vi "Send Tasks To Workers.vi"(8 "error in (no error)":errorcluster, 11 "BuildServer in":refnum<class "BuildServer.lvclass">) -> (0 "error out":errorcluster, 3 "BuildServer out":refnum<class "BuildServer.lvclass">)   [LabVIEW 2017, in "BuildServer.lvlib" / "BuildServer.lvclass"]
uses:
  BuildServer.lvclass
  BuildServer.lvclass/BuildServer.ctl
  Classes/Task Interface/Task/Task.lvclass/Task.ctl
  Classes/Task Interface/Task/Read Worker.vi
  Classes/Comm Interface/Comm Interface.lvclass
  Classes/Task Interface/Task/Task.lvclass
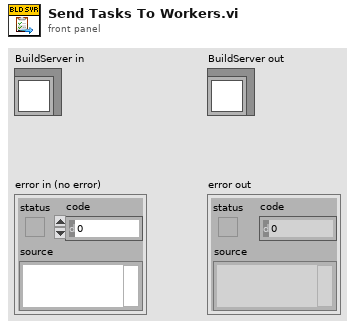
[diagram p1: front panel]
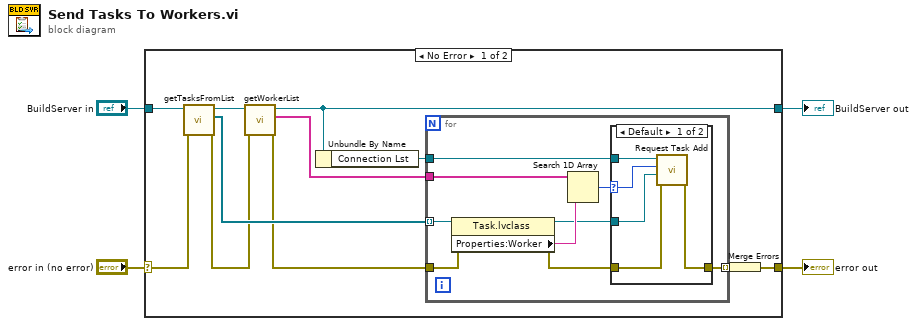
[diagram p0: block diagram]
diagram:
  n1 = case shown="No Error" "error in (no error)" {
    selector: "error in (no error)" -> [w14 w31]
    tunnel: [w5 w31] -> w3
    tunnel: [w9 w30] -> w1
    tunnel: "BuildServer in" -> [w12 w30]
    frame No Error {
      n2 = call "getTasksFromList.vi"("error in (no error)"=w14, "BuildServer in"=w12) -> ("error out"=w11:errorcluster, "Selected Tasks"=w13:refnum<class "Task.lvclass">[])  [unwired: 8 in]
      n3 = call "getWorkerList.vi"("error in (no error)"=w11, "BuildServer in"=w12) -> ("error out"=w7:errorcluster, "Worker List"=w10:string[], "BuildServer out"=w9:refnum<class "BuildServer.lvclass">)  [unwired: 7 in]
      n4 = Unbundle By Name(w9) -> ("Connection Lst"=w8:refnum<class "Comm Interface.lvclass">)
      n5 = for {
        tunnel: w13 -> [w23] mode=indexing
        tunnel: w10 -> [w22]
        tunnel: w8 -> [w18]
        tunnel: [w16] -> w6 mode=indexing
        tunnel: w7 -> [w15]
        n6 = property class="Task.lvclass"(reference=w23, error in=w15) -> (reference out=w19:refnum<class "Task.lvclass">, error out=w17:errorcluster, "Properties:Worker"=w21:string)
        n7 = Search 1D Array(1D array=w22, element=w21) -> (index of element=w20:i32)  [unwired: 1 in]
        n8 = case shown="Default" w20 {
          selector: w20 -> [w27 _]
          tunnel: w19 -> [w26 _]
          tunnel: w18 -> [w28 _]
          tunnel: w17 -> [w25 w29]
          tunnel: [w24 w29] -> w16
          frame Default {
            n9 = call "Request Task Add.vi"("error in (no error)"=w25, "Task"=w26, "index"=w27, "Comm Interface in"=w28) -> ("error out"=w24:errorcluster)  [unwired: 6 in, 1 out]
          }
          frame -1 {
          }
        }
      }
      n10 = Merge Errors(w6) -> (w5:errorcluster)
    }
    frame Error {
    }
  }
  "error out" <- w3
  "BuildServer out" <- w1
